vi "HMAC Main.vi"(2 "Secret Key":u8[](array[numeric])=[107, 101, 121], 3 "Message":u8[](array[numeric])=[84, 104, 101, 32, 113, 117, 105, 99, 107, 32, 98, 114, 111, 119, 110, 32, 102, 111, 120, 32, 106, 117, 109, 112, 115, 32, 111, 118, 101, 114, 32, 116, 104, 101, 32, 108, 97, 122, 121, 32, 100, 111, 103]) -> (0 "HMAC Out":u8[](array[numeric]) format="%x")   [LabVIEW 2014]
panel:
  # "Test Case:\n\nSecret Key: \nkey\nMessage: \nThe quick brown fox jumps over the lazy dog\n\nOutput: DE7C 9B85 B8B7 8AA6 BC8A 7A36 F70A 9070 1C9D B4D9"
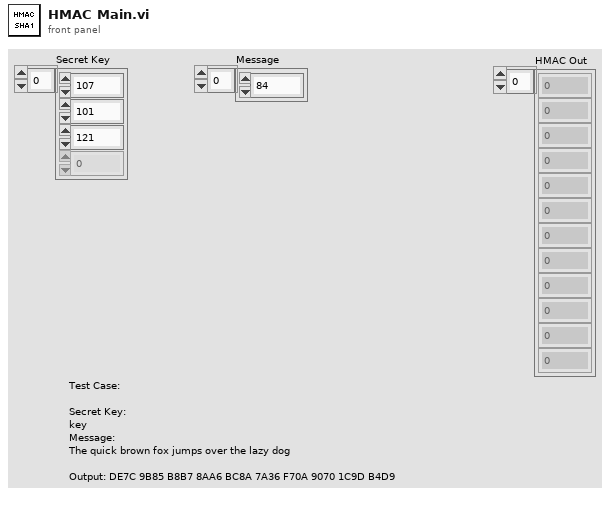
[diagram p1: front panel]
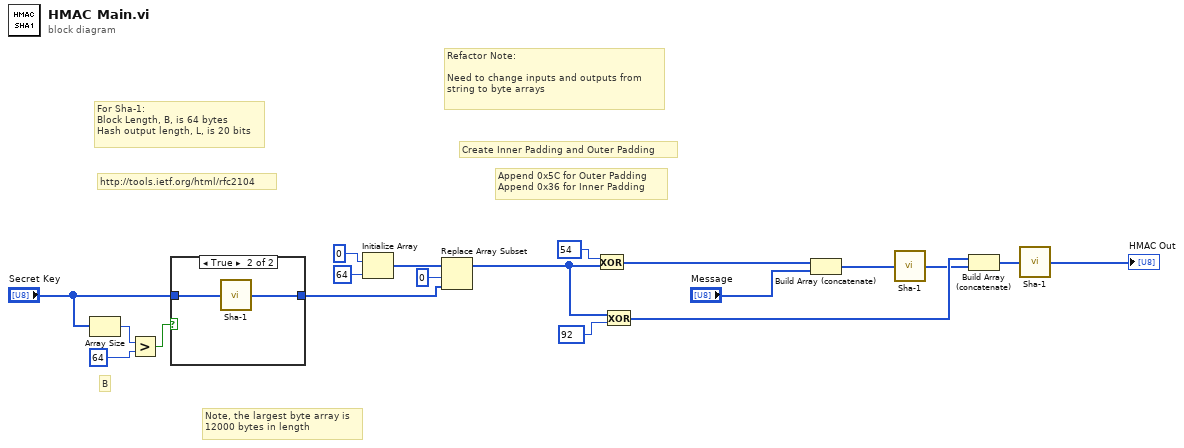
[diagram p0: block diagram]
diagram:
  # "Note, the largest byte array is \n12000 bytes in length"
  # "Refactor Note:\n\nNeed to change inputs and outputs from\nstring to byte arrays"
  # "Append 0x5C for Outer Padding\nAppend 0x36 for Inner Padding"
  # "Create Inner Padding and Outer Padding"
  # "B"
  # "http://tools.ietf.org/html/rfc2104"
  # "For Sha-1: \nBlock Length, B, is 64 bytes\nHash output length, L, is 20 bits"
  n1 = Array Size(array="Secret Key") -> (size(s)=w12:i32)
  n2 = Greater?(x=w12, y=64) -> (0:w18:bool)
  n3 = case shown="True" w18 {
    tunnel: "Secret Key" -> [w20 w22]
    tunnel: [w20 w21] -> w11
    frame False {
    }
    frame True {
      n4 = call "Sha-1.vi"("Message In as Byte Array"=w22) -> ("Digest"=w21:u8[])
    }
  }
  n5 = Initialize Array(u8 0, 64 ("dimension size")) -> (w16:u8[])
  n6 = Replace Array Subset(array=w16, new element=w11, index=0) -> (w13:u8[])
  n7 = Exclusive Or(1:w13, 2:u8 54) -> (0:w10:u8[])
  n8 = Exclusive Or(1:u8 92, 2:w13) -> (0:w8:u8[])
  n9 = Build Array (concatenate)(w10, "Message") -> (w9:u8[])
  n10 = call "Sha-1.vi"("Message In as Byte Array"=w9) -> ("Digest"=w7:u8[])
  n11 = Build Array (concatenate)(w8, w7) -> (w6:u8[])
  n12 = call "Sha-1.vi"("Message In as Byte Array"=w6) -> ("Digest"=→"HMAC Out":u8[])
